vi "TransferOption.vi"(5 "Depth":i8, 6 "Mode":u16(ring) items=["Get&Set", "Get", "Set"], 7 "Error_In":T1, 8 "Newn8BitSel":u16, 9 "ChildNo":u32, 10 "DeviceNo":u32) -> (0 "Error_Out":T1, 2 "8BitSel":u32, 3 "Error?":bool)   [LabVIEW 2015]
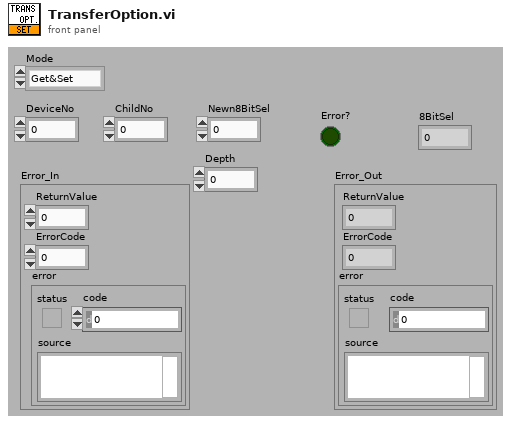
[diagram p1: front panel]
types:
  T1 = cluster{"ReturnValue":u32, "ErrorCode":u32, "error ":errorcluster}
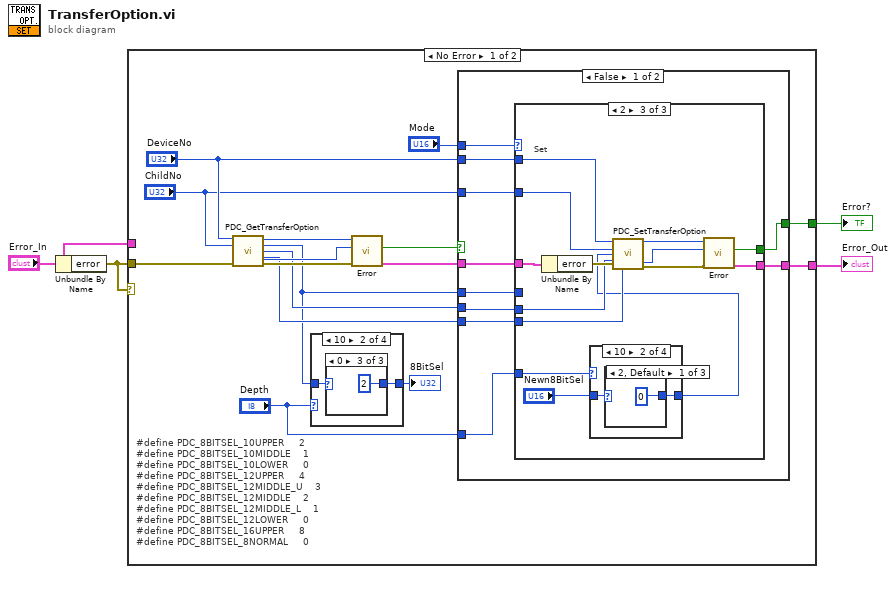
[diagram p0: block diagram]
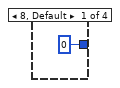
[diagram p2: hidden frame]
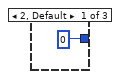
[diagram p3: hidden frame]
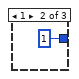
[diagram p4: hidden frame]
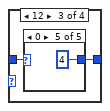
[diagram p5: hidden frame]
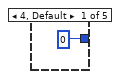
[diagram p6: hidden frame]
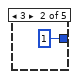
[diagram p7: hidden frame]
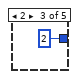
[diagram p8: hidden frame]
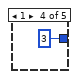
[diagram p9: hidden frame]
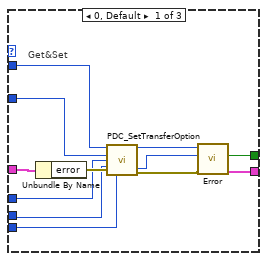
[diagram p11: hidden frame]
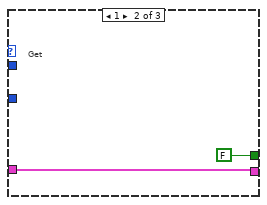
[diagram p12: hidden frame]
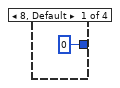
[diagram p13: hidden frame]
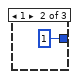
[diagram p14: hidden frame]
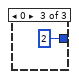
[diagram p15: hidden frame]
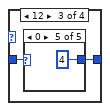
[diagram p16: hidden frame]
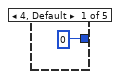
[diagram p17: hidden frame]
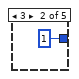
[diagram p18: hidden frame]
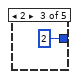
[diagram p19: hidden frame]
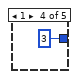
[diagram p20: hidden frame]
diagram:
  n1 = Unbundle By Name("Error_In") -> ("error"=w2:errorcluster)
  n2 = case shown="No Error" w2 {
    tunnel: [w15 w90] -> w4
    tunnel: [w12 TRUE ("Error?")] -> w3
    tunnel: w2 -> [w8 _]
    tunnel: "Error_In" -> [_ w90]
    frame No Error {
      # "#define\tPDC_8BITSEL_10UPPER\t\t\t\t\t2\n#define\tPDC_8BITSEL_10MIDDLE\t\t\t\t1\n#define\tPDC_8BITSEL_10LOWER\t\t\t\t\t0\n#define\tPDC_8BITSEL_12UPPER\t\t\t\t\t4\n#define\tPDC_8BITSEL_12MIDDLE_U\t\t\t\t3\n#define\tPDC_8BITSEL_12MIDDLE\t\t\t\t2\n#define\tPDC_8BITSEL_12MIDDLE_L\t\t\t\t1\n#define\tPDC_8BITSEL_12LOWER\t\t\t\t\t0\n#define\tPDC_8BITSEL_16UPPER\t\t\t\t\t8\n#define\tPDC_8BITSEL_8NORMAL\t\t\t\t\t0"
      n3 = call "PDC_GetTransferOption.vi"("DeviceNo"="DeviceNo", "ChildNo"="ChildNo", "error in (no error)"=w8) -> ("ReturnValue"=w19:u32, "8BitSel"=w7:u32, "Bayer"=w10:u32, "Interleave"=w9:u32, "ErrorCode"=w20:u32, "error out"=w18:errorcluster)  [unwired: 1 in, 6 out]
      n4 = case shown="10" "Depth" {
        tunnel: w7 -> [_ w23 w27 w34]
        tunnel: [u32 0 ("n8BitSel") w22 w28 w34] -> w6
        frame 8, Default {
        }
        frame 10 {
          n5 = case shown="0" w23 {
            tunnel: [u32 0 u32 1 u32 2] -> w22
            frame 2, Default {
            }
            frame 1 {
            }
            frame 0 {
            }
          }
        }
        frame 12 {
          n6 = case shown="0" w27 {
            tunnel: [u32 0 u32 1 u32 2 u32 3 u32 4] -> w28
            frame 4, Default {
            }
            frame 3 {
            }
            frame 2 {
            }
            frame 1 {
            }
            frame 0 {
            }
          }
        }
        frame 16 {
        }
      }
      "8BitSel" <- w6
      n7 = call "Error.vi"("error in (no error)"=w18, "ErrorCode"=w20, "ReturnValue"=w19) -> ("Error_Out"=w16:T1, "Error?"=w17:bool)  [unwired: 7 out]
      n8 = case shown="False" w17 {
        tunnel: w16 -> [w44 w88]
        tunnel: [w43 w88] -> w15
        tunnel: "DeviceNo" -> [w42 _]
        tunnel: "ChildNo" -> [w41 _]
        tunnel: [w40 TRUE ("Error?")] -> w12
        tunnel: "Mode" -> [w39 _]
        tunnel: w10 -> [w37 _]
        tunnel: w9 -> [w36 _]
        tunnel: w7 -> [w38 _]
        tunnel: "Depth" -> [w35 _]
        frame False {
          n9 = case shown="2" w39 {
            tunnel: w44 -> [w56 w58 w72]
            tunnel: [w51 w58 w67] -> w43
            tunnel: w42 -> [w50 _ w66]
            tunnel: w41 -> [w49 _ w65]
            tunnel: [w48 FALSE ("Error?") w64] -> w40
            tunnel: w38 -> [w45 _ _]
            tunnel: w37 -> [w46 _ w63]
            tunnel: w36 -> [w47 _ w62]
            tunnel: w35 -> [_ _ w59]
            frame 0, Default {
              # "Get&Set"
              n10 = Unbundle By Name(w56) -> ("error"=w55:errorcluster)
              n11 = call "PDC_SetTransferOption.vi"("DeviceNo"=w50, "ChildNo"=w49, "8BitSel"=w45, "Bayer"=w46, "error in (no error)"=w55, "Interleave"=w47) -> ("ReturnValue"=w54:u32, "ErrorCode"=w53:u32, "error out"=w52:errorcluster)  [unwired: 7 out]
              n12 = call "Error.vi"("error in (no error)"=w52, "ErrorCode"=w53, "ReturnValue"=w54) -> ("Error_Out"=w51:T1, "Error?"=w48:bool)  [unwired: 7 out]
            }
            frame 1 {
              # "Get"
            }
            frame 2 {
              # "Set"
              n13 = Unbundle By Name(w72) -> ("error"=w71:errorcluster)
              n14 = case shown="10" w59 {
                tunnel: "Newn8BitSel" -> [_ w75 w79 w86]
                tunnel: [u32 0 ("n8BitSel") w74 w80 w86] -> w61
                frame 8, Default {
                }
                frame 10 {
                  n15 = case shown="2, Default" w75 {
                    tunnel: [u32 0 u32 1 u32 2] -> w74
                    frame 2, Default {
                    }
                    frame 1 {
                    }
                    frame 0 {
                    }
                  }
                }
                frame 12 {
                  n16 = case shown="0" w79 {
                    tunnel: [u32 0 u32 1 u32 2 u32 3 u32 4] -> w80
                    frame 4, Default {
                    }
                    frame 3 {
                    }
                    frame 2 {
                    }
                    frame 1 {
                    }
                    frame 0 {
                    }
                  }
                }
                frame 16 {
                }
              }
              n17 = call "PDC_SetTransferOption.vi"("DeviceNo"=w66, "ChildNo"=w65, "8BitSel"=w61, "Bayer"=w63, "error in (no error)"=w71, "Interleave"=w62) -> ("ReturnValue"=w70:u32, "ErrorCode"=w69:u32, "error out"=w68:errorcluster)  [unwired: 7 out]
              n18 = call "Error.vi"("error in (no error)"=w68, "ErrorCode"=w69, "ReturnValue"=w70) -> ("Error_Out"=w67:T1, "Error?"=w64:bool)  [unwired: 7 out]
            }
          }
        }
        frame True {
        }
      }
    }
    frame Error {
    }
  }
  "Error_Out" <- w4
  "Error?" <- w3
